vi "sql-writeinfo_vproject.vi"(0 "input-IP":string="sql2012agl01.luxshare.com.cn", 1 "input-user":string="htpsuser", 2 "input-psw":string="htps'songyy", 3 "input-db":string="HTPSDB", 4 "操作模式":enum16{"写入数据", "更改数据"}(ring), 6 "表名":string="vproject", 7 "列名":string[](array[string])=["LuxsharePN", "CustomerPN", "Customer", "ProjectName", "SampleDes", "AWG", "Length", "LimitSpec", "SwitchMatrix", "EEPROMWrite", "EEPROMContent", "LabelPrint", "LabelContent", "Remarks"], 8 "DBSet":T1, 9 "值":string[](array[string]), 11 "设置":string, 13 "条件":string) -> (12 "简单报错":string, 15 "status":bool)   [LabVIEW 2011]
panel:
  out "具体错误":string
  out "字符串":string
  out "错误输出 2":errorcluster caption="错误输出"
  out "code":i32
  out "错误输出":errorcluster
  in  "ADODB._Recordset":refnum<k7>
  in  "ADODB._Connection":refnum<k7>
  # "输       入"
  # "输       出"
  # "写入数据，需要指定写入列的名称，以及与之对应的值"
  # "基本信息\n（）"
  # "状态灯，False表示操作成功，True表示操作失败"
  # "错误信息"
  # "改变操作时需要修改的信息"
  # "操作模式：写入数据\n                  更改数据"
  # "表名"
  # "更改数据，需要指定修改列的新值"
  # "更改数据，利用条件找到需要修改的行"
  # "error:\n-2147217843 登陆失败： 。\n-2147467259 要访问的数据库不存在\n-2146825267 没有数据    。\n-2146824584 对象关闭时，不允许操作\n-2147217865 表名不存在 。\n-2147467259 服务器连接失败 。\n-2147217900 列名无效\n-2147217900 不允许有NULL值\n-2147217900 unique的键重复"
  # "error:\n-2147217900 所创建的表已经存在\n-2147217900 该列不存在"
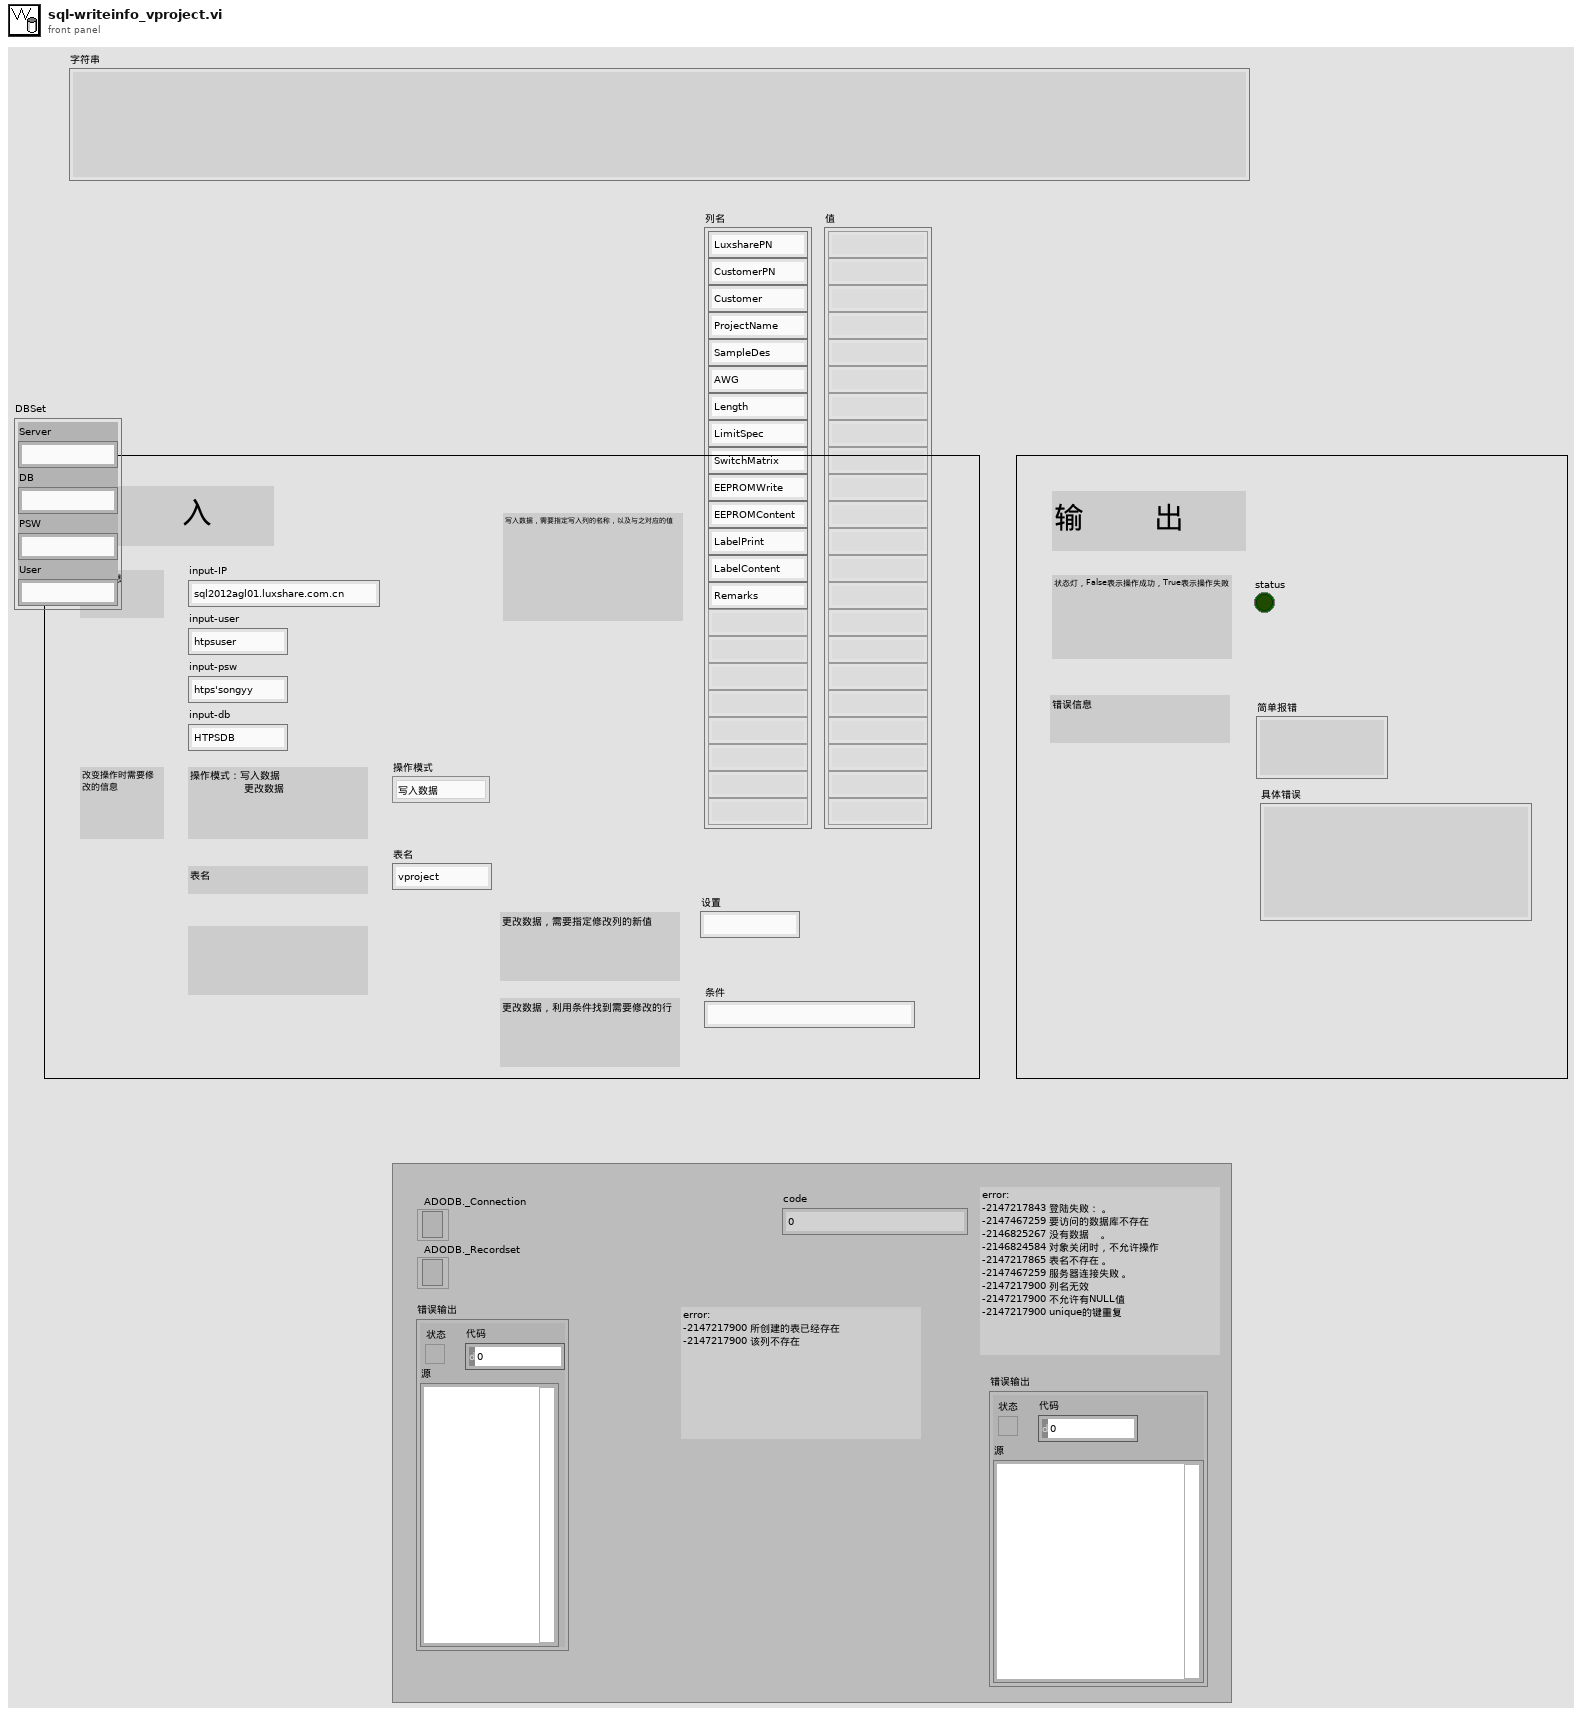
[diagram p1: front panel]
types:
  T1 = cluster{"Server":string, "DB":string, "PSW":string, "User":string}
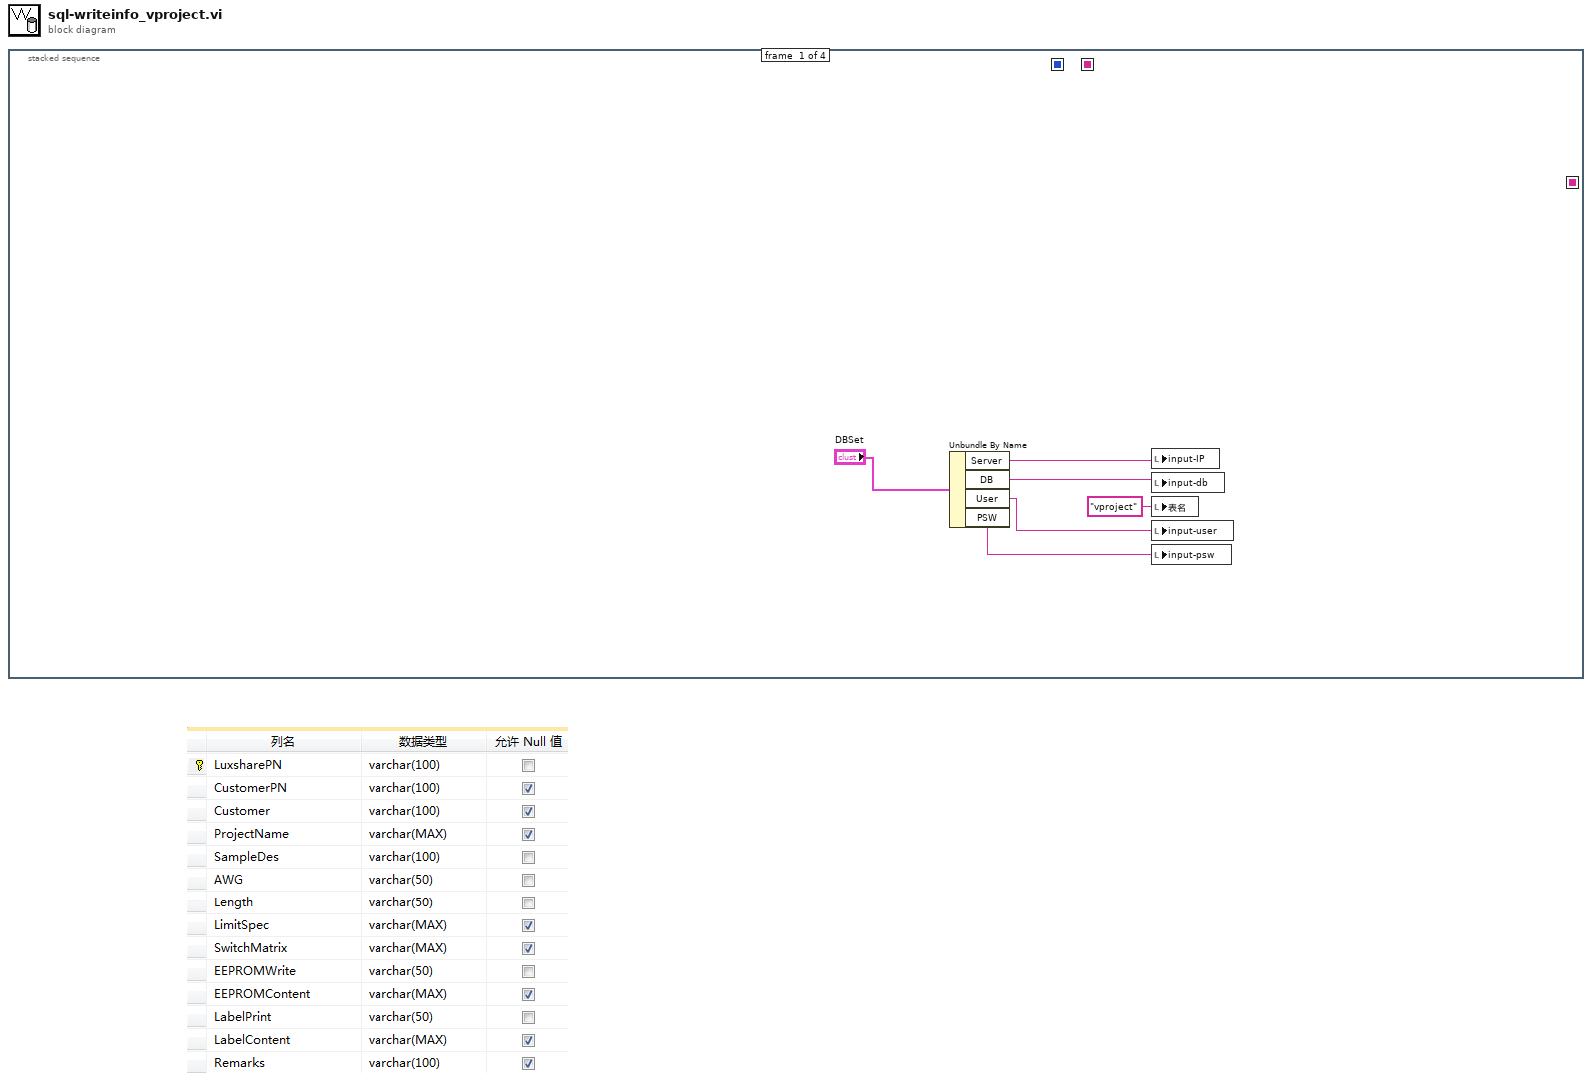
[diagram p0: block diagram]
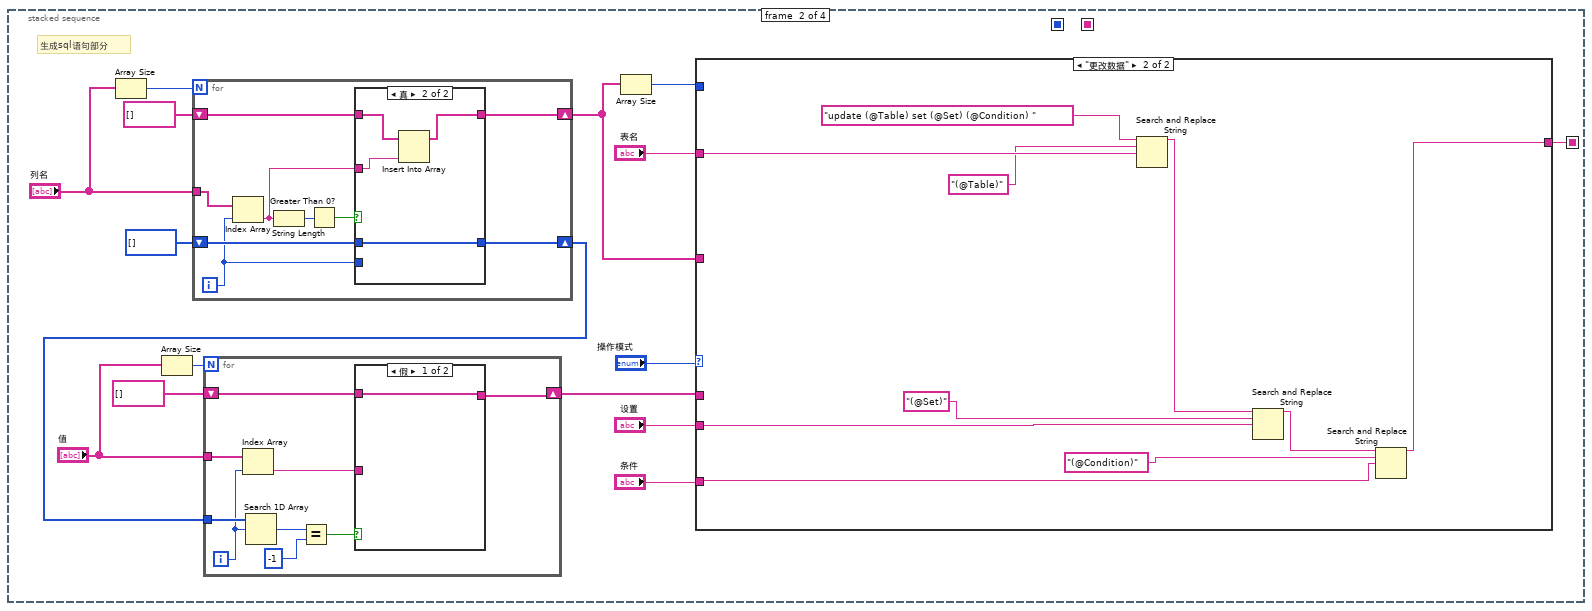
[diagram p2: hidden frame]
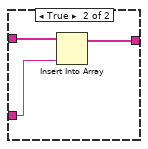
[diagram p3: hidden frame]
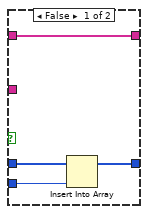
[diagram p4: hidden frame]
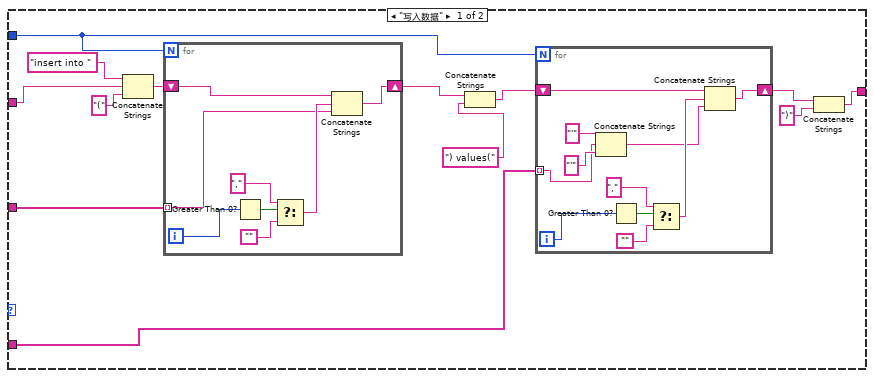
[diagram p5: hidden frame]
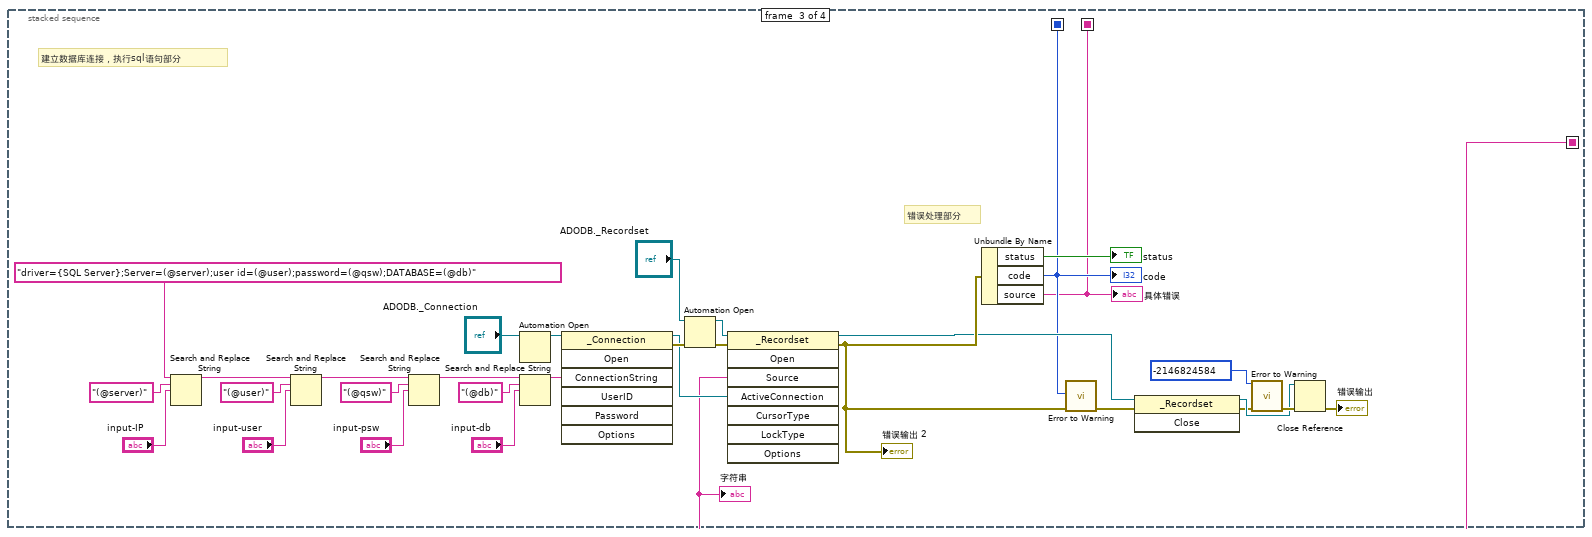
[diagram p6: hidden frame]
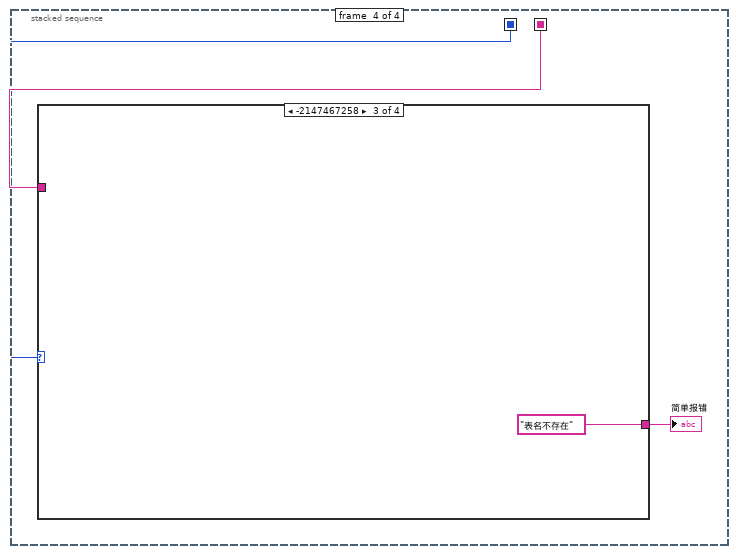
[diagram p7: hidden frame]
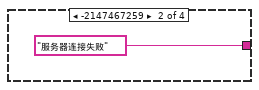
[diagram p9: hidden frame]
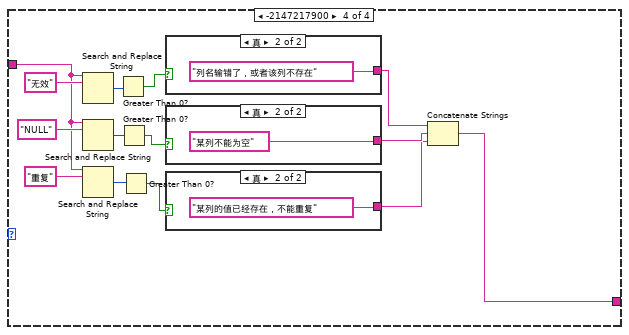
[diagram p10: hidden frame]
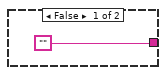
[diagram p11: hidden frame]
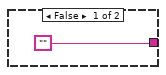
[diagram p12: hidden frame]
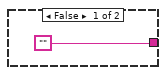
[diagram p13: hidden frame]
diagram:
  n1 = stacked-sequence {
    seq-local: [_ w7 _ _] -> [_ _ w98 _]
    seq-local: [_ _ w96 _] -> [_ _ _ w128]
    seq-local: [_ _ w95 _] -> [_ _ _ w127]
    frame #0 {
      n2 = Unbundle By Name("DBSet") -> ("Server"=w5:string, "DB"=w4:string, "User"=w3:string, "PSW"=w2:string)
      n3 = local write "input-IP"(w5) -> ()
      n4 = local write "input-db"(w4) -> ()
      n5 = local write "表名"("vproject" ("表名")) -> ()
      n6 = local write "input-user"(w3) -> ()
      n7 = local write "input-psw"(w2) -> ()
    }
    frame #1 {
      # "生成sql语句部分"
      n8 = Array Size(array="列名") -> (size(s)=w19:i32)
      n9 = Array Size(array="值") -> (size(s)=w16:i32)
      n10 = for {
        N: w19 -> [_]
        tunnel: "列名" -> [w44]
        shift-right: [w39] -> w11
        shift-left: string[] [] -> [w40]
        shift-right: [w36] -> w14
        shift-left: i32[] [] -> [w38]
        i -> [w37]
        n11 = Index Array(array=w44, index=w37) -> (element=w41:string)
        n12 = String Length(string=w41) -> (length=w43:i32)
        n13 = Greater Than 0?(x=w43) -> (x > 0?=w42:bool)
        n14 = case shown="真" w42 {
          tunnel: w41 -> [_ w50]
          tunnel: w40 -> [w48 w52]
          tunnel: [w48 w51] -> w39
          tunnel: w38 -> [w47 w49]
          tunnel: w37 -> [w46 _]
          tunnel: [w45 w49] -> w36
          frame False {
            n15 = Insert Into Array(array=w47, new element=w46) -> (w45:i32[])  [unwired: 1 in]
          }
          frame True {
            n16 = Insert Into Array(array=w52, new element=w50) -> (w51:string[])  [unwired: 1 in]
          }
        }
      }
      n17 = for {
        N: w16 -> [_]
        shift-right: [w23] -> w10
        shift-left: string[] [] -> [w24]
        tunnel: "值" -> [w28]
        tunnel: w14 -> [w31]
        i -> [w27]
        n18 = Index Array(array=w28, index=w27) -> (element=w25:string)
        n19 = Search 1D Array(1D array=w31, element=w27) -> (index of element=w30:i32)  [unwired: 1 in]
        n20 = Equal?(x=w30, y=-1) -> (x = y?=w26:bool)
        n21 = case shown="假" w26 {
          tunnel: w25 -> [_ w33]
          tunnel: w24 -> [w32 w35]
          tunnel: [w32 w34] -> w23
          frame False {
          }
          frame True {
            n22 = Insert Into Array(array=w35, new element=w33) -> (w34:string[])  [unwired: 1 in]
          }
        }
      }
      n23 = Array Size(array=w11) -> (size(s)=w20:i32)
      n24 = case shown="\"更改数据\"" "操作模式" {
        tunnel: "表名" -> [w65 w92]
        tunnel: [w56 w85] -> w7
        tunnel: w20 -> [w62 _]
        tunnel: w11 -> [w53 _]
        tunnel: w10 -> [w55 _]
        tunnel: "设置" -> [_ w94]
        tunnel: "条件" -> [_ w86]
        frame "写入数据" {
          n25 = Concatenate Strings("insert into ", w65, "(") -> (w63:string)
          n26 = for {
            N: w62 -> [_]
            shift-right: [w78] -> w61
            shift-left: w63 -> [w84]
            tunnel: w53 -> [w79] mode=indexing
            i -> [w77]
            n27 = Greater Than 0?(x=w77) -> (x > 0?=w83:bool)
            n28 = Select(t=",", s=w83, f="") -> (s? t:f=w80:string)
            n29 = Concatenate Strings(w84, w80, w79) -> (w78:string)
          }
          n30 = Concatenate Strings(w61, ") values(") -> (w59:string)
          n31 = for {
            N: w62 -> [_]
            shift-right: [w70] -> w58
            shift-left: w59 -> [w76]
            tunnel: w55 -> [w67] mode=indexing
            i -> [w75]
            n32 = Concatenate Strings("'", w67, "'") -> (w66:string)
            n33 = Greater Than 0?(x=w75) -> (x > 0?=w74:bool)
            n34 = Select(t=",", s=w74, f="") -> (s? t:f=w71:string)
            n35 = Concatenate Strings(w76, w71, w66) -> (w70:string)
          }
          n36 = Concatenate Strings(w58, ")") -> (w56:string)
        }
        frame "更改数据" {
          n37 = Search and Replace String(input string="update (@Table) set (@Set) (@Condition) ", search string="(@Table)", replace string=w92) -> (result string=w89:string)  [unwired: 5 in, 3 out]
          n38 = Search and Replace String(input string=w89, search string="(@Set)", replace string=w94) -> (result string=w88:string)  [unwired: 5 in, 3 out]
          n39 = Search and Replace String(input string=w88, search string="(@Condition)", replace string=w86) -> (result string=w85:string)  [unwired: 5 in, 3 out]
        }
      }
    }
    frame #2 {
      # "错误处理部分"
      # "建立数据库连接，执行sql语句部分"
      n40 = Search and Replace String(input string="driver={SQL Server};Server=(@server);user id=(@user);password=(@qsw);DATABASE=(@db)" ("ConnectionString"), search string="(@server)" ("搜索字符串"), replace string="input-IP") -> (result string=w103:string)  [unwired: 5 in, 3 out]
      n41 = Search and Replace String(input string=w103, search string="(@user)" ("搜索字符串"), replace string="input-user") -> (result string=w106:string)  [unwired: 5 in, 3 out]
      n42 = Search and Replace String(input string=w106, search string="(@qsw)" ("搜索字符串"), replace string="input-psw") -> (result string=w109:string)  [unwired: 5 in, 3 out]
      n43 = Automation Open(Automation Refnum="ADODB._Connection") -> (Automation Refnum=w99:refnum<k7>)  [unwired: 3 in, 1 out]
      n44 = Search and Replace String(input string=w109, search string="(@db)" ("搜索字符串"), replace string="input-db") -> (result string=w113:string)  [unwired: 5 in, 3 out]
      n45 = invoke class="_Connection" method="Open"(reference=w99, "ConnectionString"=w113) -> (reference out=w115:refnum<k7>, error out=w117:errorcluster)  [unwired: 5 in, 5 out]
      n46 = Automation Open(error in (no error)=w117, Automation Refnum="ADODB._Recordset") -> (Automation Refnum=w116:refnum<k7>, error out=w118:errorcluster)  [unwired: 2 in]
      n47 = invoke class="_Recordset" method="Open"(reference=w116, error in=w118, "Source"=w98, "ActiveConnection"=w115) -> (reference out=w125:refnum<k7>, error out=w126:errorcluster)  [unwired: 4 in, 6 out]
      "错误输出 2" <- w126
      n48 = Unbundle By Name(w126) -> ("status"=→"status":bool, "code"=w96:i32, "source"=w95:string)
      "code" <- w96
      "具体错误" <- w95
      n49 = call <vilib>:"Error to Warning.vi"("1st Error to Convert"=w96, "error in"=w126) -> ("warning out"=w119:errorcluster)  [unwired: 13 in]
      n50 = invoke class="_Recordset" method="Close"(reference=w125, error in=w119) -> (reference out=w123:refnum<k7>, error out=w120:errorcluster)  [unwired: 1 in, 1 out]
      n51 = call <vilib>:"Error to Warning.vi"("1st Error to Convert"=-2146824584, "error in"=w120) -> ("warning out"=w124:errorcluster)  [unwired: 13 in]
      n52 = Close Reference(reference=w123, error in (no error)=w124) -> (error out=→"错误输出":errorcluster)
      "字符串" <- w98
    }
    frame #3 {
      n53 = case shown="-2147467258" w128 {
        tunnel: [_ "服务器连接失败" "表名不存在" w132] -> w129
        tunnel: w127 -> [_ _ _ w143]
        frame 0, Default {
        }
        frame -2147467259 {
        }
        frame -2147467258 {
        }
        frame -2147217900 {
          n54 = Search and Replace String(input string=w143, search string="无效" ("搜索字符串")) -> (number of replacements=w141:i32)  [unwired: 6 in, 3 out]
          n55 = Search and Replace String(input string=w143, search string="NULL" ("搜索字符串")) -> (number of replacements=w140:i32)  [unwired: 6 in, 3 out]
          n56 = Search and Replace String(input string=w143, search string="重复" ("搜索字符串")) -> (number of replacements=w139:i32)  [unwired: 6 in, 3 out]
          n57 = Greater Than 0?(x=w141) -> (x > 0?=w138:bool)
          n58 = Greater Than 0?(x=w140) -> (x > 0?=w137:bool)
          n59 = Greater Than 0?(x=w139) -> (x > 0?=w136:bool)
          n60 = case shown="真" w138 {
            tunnel: ["" "列名输错了，或者该列不存在"] -> w135
            frame False {
            }
            frame True {
            }
          }
          n61 = case shown="真" w137 {
            tunnel: ["" "某列不能为空"] -> w134
            frame False {
            }
            frame True {
            }
          }
          n62 = case shown="真" w136 {
            tunnel: ["" "某列的值已经存在，不能重复"] -> w133
            frame False {
            }
            frame True {
            }
          }
          n63 = Concatenate Strings(w135, w134, w133) -> (w132:string)
        }
      }
      "简单报错" <- w129
    }
  }
